vi "WPI_DMAAddChannelToStream_DigitalInput.vi"(7 "DigitalInputDevRef":T1={"DevStatus"={"status"=FALSE, "code"=0, "source"=""}, "DIO Channel"=enum."DIO 1"}, 8 "error in (no error)":errorcluster, 10 "Digital Input Type":T3, 11 "DMARef":T4) -> (0 "error out":errorcluster, 3 "DMARef":T4)   [LabVIEW 2017]
doc: "Specifies the data transferred in the DMA stream. Wire a device reference from the other WPI Robotics Library Open VIs to specify the data you want to receive. The order that the AddChannel VIs add data to the DMA stream defines the order that the Read VI returns the data.\n\nSpecifies the digital input data transferred in the DMA stream.\n\nYou must open a reference to a DMA stream with the Open VI before using this VI.\n\nThis software is licensed. Open the labview\\readme\\WPI Robotics Library Open Source License.txt file for more information."
uses:
  <vilib>/Rock Robotics/WPI/DMA/WPI_DMARef.ctl
  <vilib>/Rock Robotics/WPI/DMA/WPI_DMADigitalInputType.ctl
  <vilib>/Rock Robotics/WPI/DigitalInput/WPI_DigitalInputDevRef.ctl
  <vilib>/Rock Robotics/SystemInterfaces/DIO/FPGA_DIOChannel.ctl
  <vilib>/Rock Robotics/WPI/DMA/WPI_DMAChannelTypeEnum.ctl
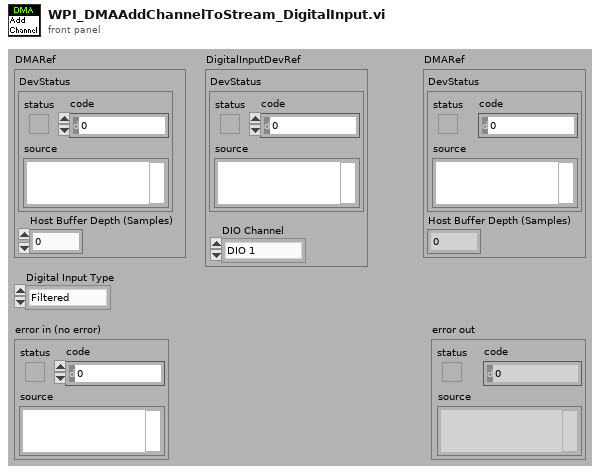
[diagram p1: front panel]
types:
  T1 = typedef "WPI_DigitalInputDevRef.ctl" = cluster{"DevStatus":errorcluster, "DIO Channel":T2}
  T2 = typedef "FPGA_DIOChannel.ctl" = enum8{"DIO 0", "DIO 1", "DIO 2", "DIO 3", "DIO 4", "DIO 5", "DIO 6", "DIO 7", "DIO 8", "DIO 9", "DIO MXP 0", "DIO MXP 1", "DIO MXP 2", "DIO MXP 3", "DIO MXP 4", "DIO MXP 5", "DIO MXP 6", "DIO MXP 7", "DIO MXP 8", "DIO MXP 9", "DIO MXP 10", "DIO MXP 11", "DIO MXP 12", "DIO MXP 13", "DIO MXP 14", "DIO MXP 15", "SPI Port CS1", "SPI Port CS2", "SPI Port CS3", "SPI Port MISO", "SPI Port MOSI", "Invalid"}
  T3 = typedef "WPI_DMADigitalInputType.ctl" = enum16{"Filtered", "Raw"}
  T4 = typedef "WPI_DMARef.ctl" = cluster{"DevStatus":errorcluster, "Host Buffer Depth (Samples)":u32}
  T5 = typedef "WPI_DMAChannelTypeEnum.ctl" = enum16{"AI (Raw)", "AI (Avg)", "Accumulator", "DI (Raw) Onboard", "DI (Filtered) Onboard", "DI (Raw) MXP", "DI (Filtered) MXP", "Analog Trigger", "Counter", "Counter (Timer)", "Encoder", "Encoder (Timer)", "Time Stamp"}
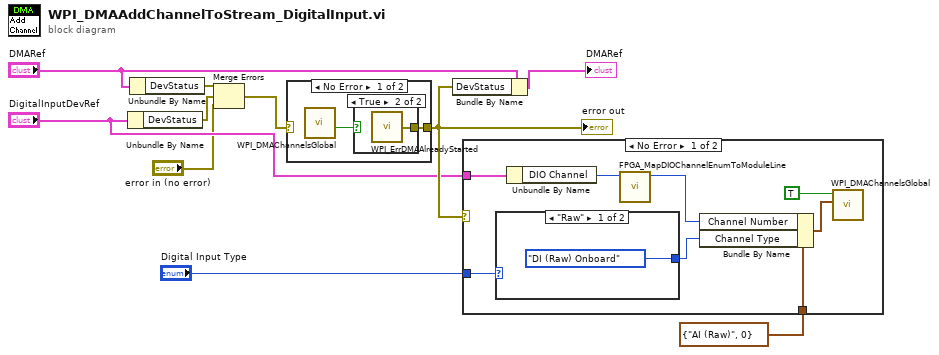
[diagram p0: block diagram]
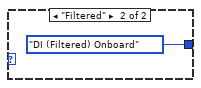
[diagram p2: hidden frame]
diagram:
  n1 = Unbundle By Name("DigitalInputDevRef") -> ("DevStatus"=w3:errorcluster)
  n2 = Unbundle By Name("DMARef") -> ("DevStatus"=w4:errorcluster)
  n3 = Merge Errors(w4, w3, "error in (no error)") -> (w1:errorcluster)
  n4 = case shown="No Error" w1 {
    selector: w1 -> [_ w14]
    tunnel: [w11 w14] -> w9
    frame No Error {
      n5 = call <vilib>:"WPI_DMAChannelsGlobal.vi"() -> ("Started"=w12:bool)  [unwired: 4 in, 7 out]
      n6 = case shown="True" w12 {
        tunnel: [_ w13] -> w11
        frame False {
        }
        frame True {
          n7 = call <vilib>:"WPI_ErrDMAAlreadyStarted.vi"() -> ("error out"=w13:errorcluster)
        }
      }
    }
    frame Error {
    }
  }
  "error out" <- w9
  n8 = Bundle By Name(cluster="DMARef", "DevStatus"=w9) -> (→"DMARef":T4)
  n9 = case shown="No Error" w9 {
    tunnel: "DigitalInputDevRef" -> [w21 _]
    tunnel: cluster{"Channel Type":T5, "Channel Number":u8} {"Channel Type"=enum."AI (Raw)", "Channel Number"=0} ("Channel") -> [w19 _]
    tunnel: "Digital Input Type" -> [w16 _]
    frame No Error {
      n10 = case shown="\"Raw\"" w16 {
        tunnel: [WPI_DMAChannelTypeEnum."DI (Raw) Onboard" ("Channel Type") WPI_DMAChannelTypeEnum."DI (Filtered) Onboard" ("Channel Type")] -> w18
        frame "Raw" {
        }
        frame "Filtered" {
        }
      }
      n11 = Unbundle By Name(w21) -> ("DIO Channel"=w20:T2)
      n12 = call <vilib>:"FPGA_MapDIOChannelEnumToModuleLine.vi"("DIOChannel"=w20) -> ("ActualDIOChannel(U8)"=w17:u8)  [unwired: 10 out]
      n13 = Bundle By Name(cluster=w19, "Channel Number"=w17, "Channel Type"=w18) -> (w15:cluster{"Channel Type":T5, "Channel Number":u8})
      n14 = call <vilib>:"WPI_DMAChannelsGlobal.vi"("Channel"=w15, "Add"=TRUE) -> ()  [unwired: 2 in, 8 out]
    }
    frame Error {
    }
  }
